vi "IT8800-Query Range.vi"(8 "error in":errorcluster, 10 "Range Type":u16(ring) items=["Current", "Voltage", "Power", "Resistance"], 11 "IT8800 Setting In In":T1={"VISA Resource Name"="", "Baud Rate"=19200, "Stop Bits"=20, "Wait For Read(ms)"=0} {"Stop Bits" items=["1.0"=10, "2.0"=20]; "Baud Rate" items=["2400"=2400, "4800"=4800, "9600"=9600, "19200"=19200]}) -> (0 "error out":errorcluster, 2 "Range":u16(ring)=2 items=["Low", "Medium", "High"], 3 "IT8800 Setting In Out":T1={"VISA Resource Name"="", "Baud Rate"=19200, "Stop Bits"=20, "Wait For Read(ms)"=0} {"Stop Bits" items=["1.0"=10, "2.0"=20]; "Baud Rate" items=["2400"=2400, "4800"=4800, "9600"=9600, "19200"=19200]})   [LabVIEW 2018]
uses:
  Data Def/IT8800-Setting.ctl
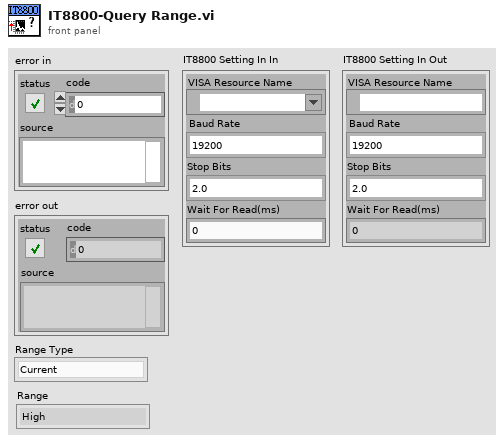
[diagram p1: front panel]
types:
  T1 = typedef "IT8800-Setting.ctl" = cluster{"VISA Resource Name":refnum<visa-resource-name>, "Baud Rate":u32, "Stop Bits":u16, "Wait For Read(ms)":u32}
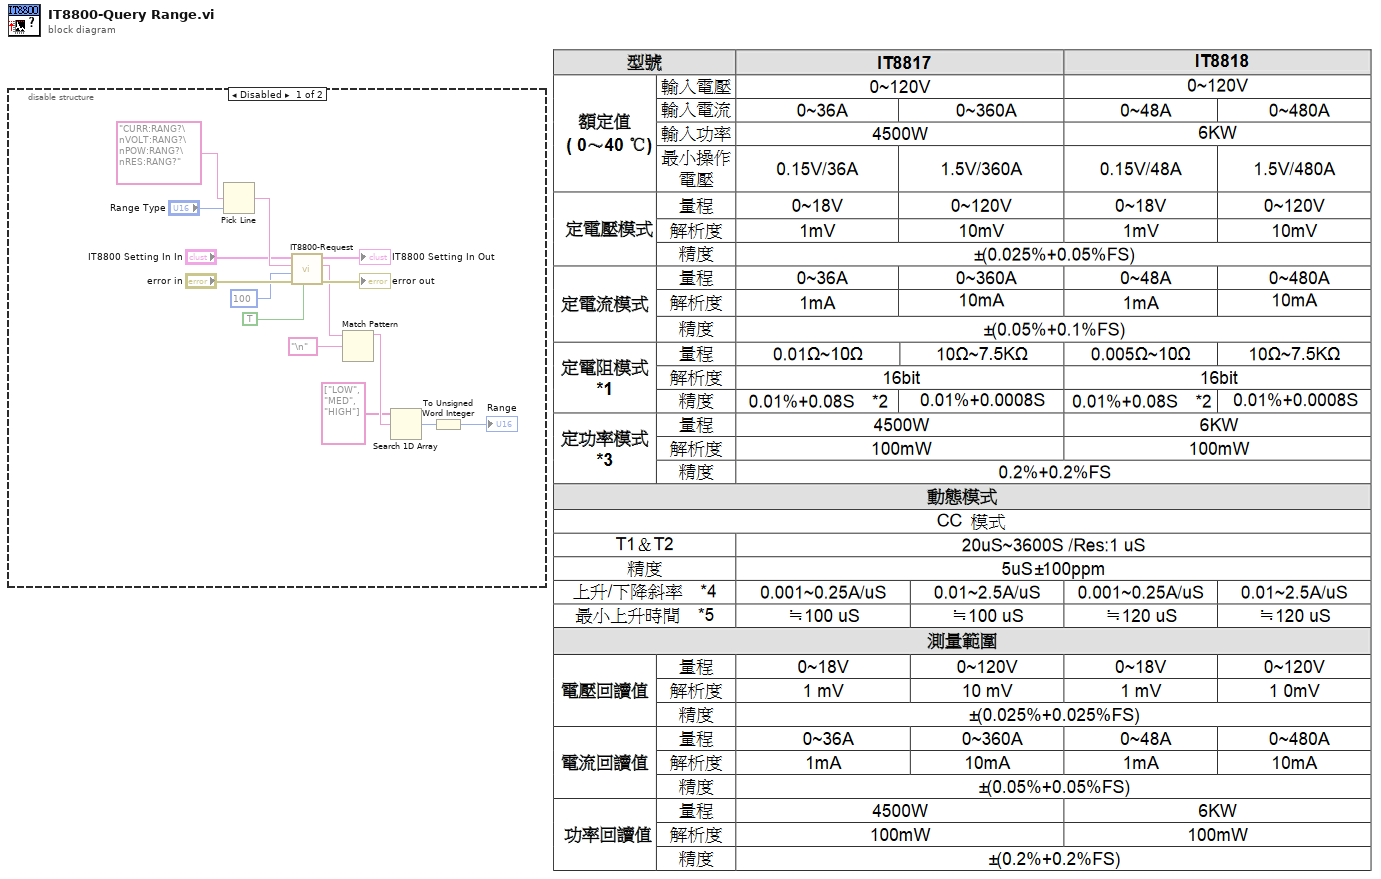
[diagram p0: block diagram]
diagram:
  n1 = disable-structure shown="Disabled" {
    frame Disabled {
      n2 = Pick Line(multi-line string="CURR:RANG?\nVOLT:RANG?\nPOW:RANG?\nRES:RANG?", line index="Range Type") -> (output string=w9:string)  [unwired: 1 in]
      n3 = call "IT8800-Request.vi"("Response?"=TRUE, "error in"="error in", "byte count"=u32 100, "Command"=w9, "IT8800 Setting In In"="IT8800 Setting In In") -> ("error out"=→"error out":errorcluster, "Response"=w8:string, "IT8800 Setting In Out"=→"IT8800 Setting In Out":T1)  [unwired: 4 in]
      n4 = Match Pattern(string=w8, regular expression="\n") -> (before substring=w6:string)  [unwired: 1 in, 3 out]
      n5 = Search 1D Array(1D array=string[] ["LOW", "MED", "HIGH"], element=w6) -> (index of element=w4:i32)  [unwired: 1 in]
      n6 = To Unsigned Word Integer(number=w4) -> (unsigned 16bit integer=→"Range":u16)
    }
    frame Enabled {
    }
  }
